vi "Default Database.vi"(8 "error in":errorcluster) -> (0 "error out":errorcluster, 3 "DB":T1)   [LabVIEW 2010, in "Config Database.lvlib"]
doc: "This VI enqueues the named action."
uses:
  Config Database.lvlib
  Private Controls/DB Data.ctl
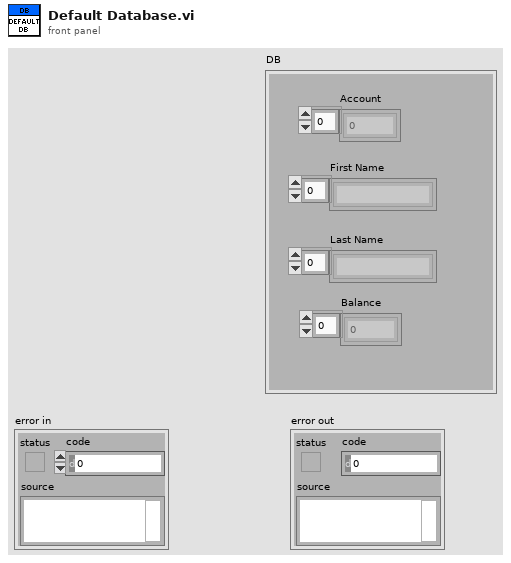
[diagram p1: front panel]
types:
  T1 = typedef "Config Database.lvlib/DB Data.ctl" = cluster{"Account":dbl[], "First Name":string[], "Last Name":string[], "Balance":dbl[]}
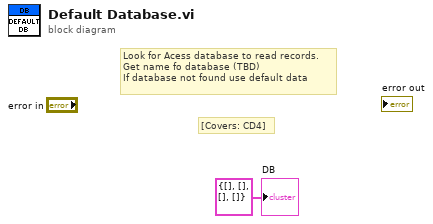
[diagram p0: block diagram]
diagram:
  # "[Covers: CD4]"
  # "Look for Acess database to read records.\nGet name fo database (TBD)\nIf database not found use default data"
  "DB" <- T1 {"Account"=[], "First Name"=[], "Last Name"=[], "Balance"=[]} ("DB")
